vi "Variant_Extraction.vi"(8 "error in":errorcluster, 11 "Input cluster":cluster{"String":string, "Value":variant}) -> (0 "error out":errorcluster, 2 "Output cluster":T1, 3 "type":T2)   [LabVIEW 2024]
uses:
  <vilib>/Utility/Data Type/Type Definitions/Data Type.ctl
  <vilib>/Utility/Data Type/NI_Data Type.lvlib
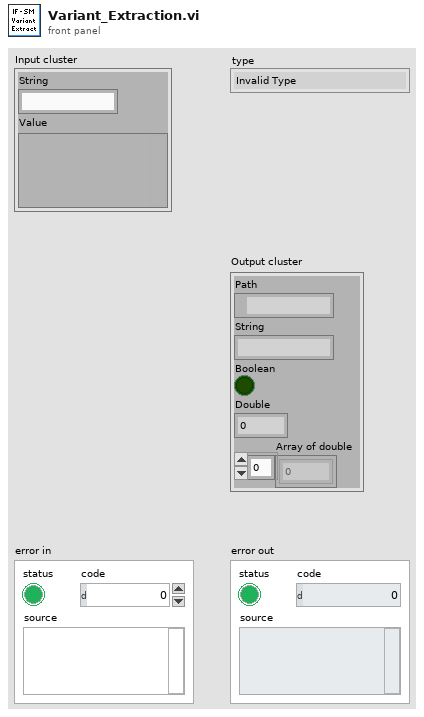
[diagram p1: front panel]
types:
  T1 = cluster{"Path":path, "String":string, "Boolean":bool, "Double":dbl, "Array of double":dbl[]}
  T2 = typedef "NI_Data Type.lvlib/Data Type.ctl" = enum8{"Invalid Type", "Void", "I8", "I16", "I32", "I64", "U8", "U16", "U32", "U64", "Single Float", "Double Float", "Extended Float", "Single Complex", "Double Complex", "Extended Complex", "Enum U8", "Enum U16", "Enum U32", "Enum U64", "Single Float With Unit", "Double Float With Unit", "Extended Float With Unit", "Single Complex with Unit", "Double Complex with Unit", "Extended Complex with Unit", "Boolean", "String", "Path", "Picture", "Tag", "Array", "Cluster", "Variant", "LV Variant", "Waveform", "Timestamp", "Digital Waveform", "Digital Data", "ExpressData", "Refnum", "External Data", "VI", "Poly VI", "LabVIEW Class Instance", "Fixed Point", "Set Collection", "Map Collection"}
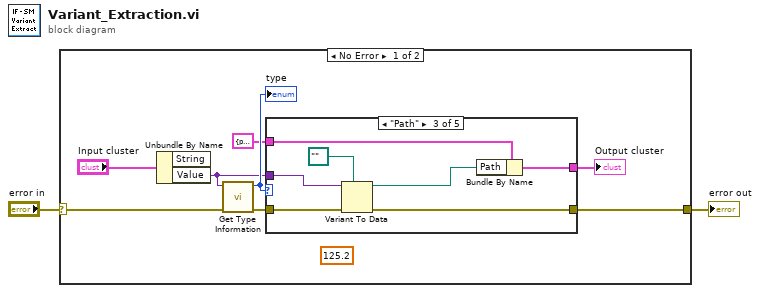
[diagram p0: block diagram]
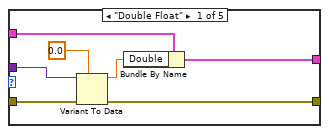
[diagram p2: hidden frame]
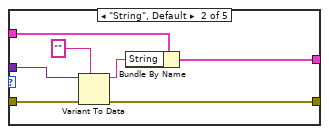
[diagram p3: hidden frame]
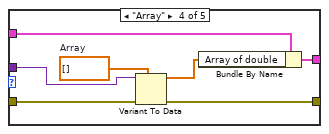
[diagram p4: hidden frame]
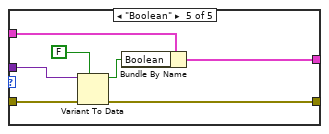
[diagram p5: hidden frame]
diagram:
  n1 = case shown="No Error" "error in" {
    selector: "error in" -> [w10 w46]
    tunnel: [w6 w46] -> w1
    frame No Error {
      (unwired) 125.2
      n2 = Unbundle By Name("Input cluster") -> ("Value"=w7:variant)  [unwired: 1 out]
      n3 = call <vilib>:"Get Type Information.vi"("error in (no error)"=w10, "variant"=w7) -> ("error out"=w8:errorcluster, "type"=w9:T2)  [unwired: 5 in, 3 out]
      "type" <- w9
      n4 = case shown="\"Path\"" w9 {
        tunnel: w8 -> [w16 w24 w31 w36 w44]
        tunnel: w7 -> [w15 w23 w29 w38 w45]
        tunnel: [w14 w21 w30 w37 w43] -> w6
        tunnel: [w12 w19 w26 w33 w39] -> w5
        tunnel: T1 {"Path"=path "", "String"="Init", "Boolean"=FALSE, "Double"=125.2, "Array of double"=[]} ("Cluster 2") -> [w11 w18 w25 w32 w40]
        frame "Double Float" {
          n5 = Variant To Data(error in=w16, type=0.0, Variant=w15) -> (data=w13:dbl, error out=w14:errorcluster)
          n6 = Bundle By Name(cluster=w11, "Double"=w13) -> (w12:T1)
        }
        frame "String", Default {
          n7 = Variant To Data(error in=w24, type="", Variant=w23) -> (data=w20:string, error out=w21:errorcluster)
          n8 = Bundle By Name(cluster=w18, "String"=w20) -> (w19:T1)
        }
        frame "Path" {
          n9 = Variant To Data(error in=w31, type=path "", Variant=w29) -> (data=w27:path, error out=w30:errorcluster)
          n10 = Bundle By Name(cluster=w25, "Path"=w27) -> (w26:T1)
        }
        frame "Array" {
          w35 = dbl[] []  # Array
          n11 = Variant To Data(error in=w36, type=w35, Variant=w38) -> (data=w34:dbl[], error out=w37:errorcluster)
          n12 = Bundle By Name(cluster=w32, "Array of double"=w34) -> (w33:T1)
        }
        frame "Boolean" {
          n13 = Variant To Data(error in=w44, type=FALSE, Variant=w45) -> (data=w41:bool, error out=w43:errorcluster)
          n14 = Bundle By Name(cluster=w40, "Boolean"=w41) -> (w39:T1)
        }
      }
      "Output cluster" <- w5
    }
    frame Error {
    }
  }
  "error out" <- w1
